vi "Refactor Classes in Project.vi"(8 "error in (no error)":errorcluster, 10 "rename data in":T1, 11 "project item in":refnum<vi>) -> (0 "error out":errorcluster, 2 "rename metadata out":T1, 3 "project item out":refnum<vi>, 4 "refactored overrides":T4[](array[typedef]), 6 "refactored classes":path[](array[path]))   [LabVIEW 2021, in "MeasurementService Editor.lvlib"]
uses:
  MeasurementService Editor.lvlib
  Rename Refactor Mapping Info.ctl
  Rename Refactor Data.ctl
  Refactor Dynamic Dispatch Member Result.ctl
  Rename String Mapping.ctl
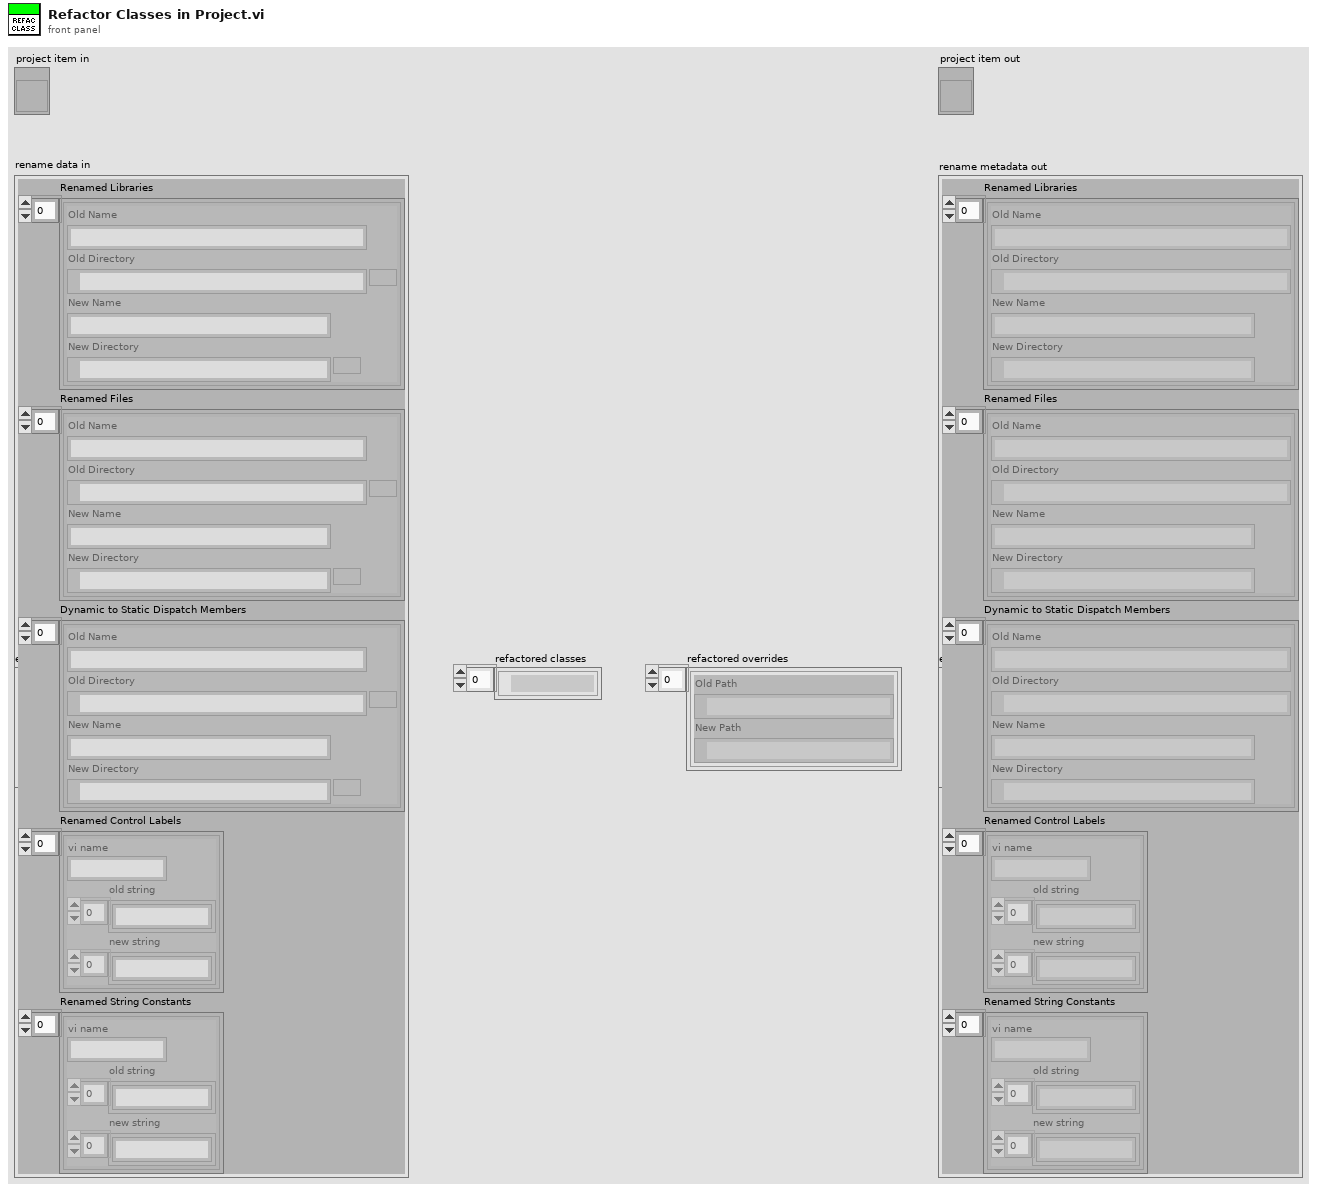
[diagram p1: front panel]
types:
  T1 = typedef "MeasurementService Editor.lvlib/Rename Refactor Data.ctl" = cluster{"Renamed Libraries":T2[], "Renamed Files":T2[], "Dynamic to Static Dispatch Members":T2[], "Renamed Control Labels":T3[], "Renamed String Constants":T3[]}
  T2 = typedef "MeasurementService Editor.lvlib/Rename Refactor Mapping Info.ctl" = cluster{"Old Name":string, "Old Directory":path, "New Name":string, "New Directory":path}
  T3 = typedef "MeasurementService Editor.lvlib/Rename String Mapping.ctl" = cluster{"vi name":string, "old string":string[], "new string":string[]}
  T4 = typedef "MeasurementService Editor.lvlib/Refactor Dynamic Dispatch Member Result.ctl" = cluster{"Old Path":path, "New Path":path}
  T5 = typedef "Copy of MeasurementService Editor.lvlib/Rename Refactor Data.ctl" = cluster{"Renamed Libraries":T6[], "Renamed Files":T6[], "Dynamic to Static Dispatch Members":T6[], "Renamed Control Labels":T7[], "Renamed String Constants":T7[]}
  T6 = typedef "Copy of MeasurementService Editor.lvlib/Rename Refactor Mapping Info.ctl" = cluster{"Old Name":string, "Old Directory":path, "New Name":string, "New Directory":path}
  T7 = typedef "Copy of MeasurementService Editor.lvlib/Rename String Mapping.ctl" = cluster{"vi name":string, "old string":string[], "new string":string[]}
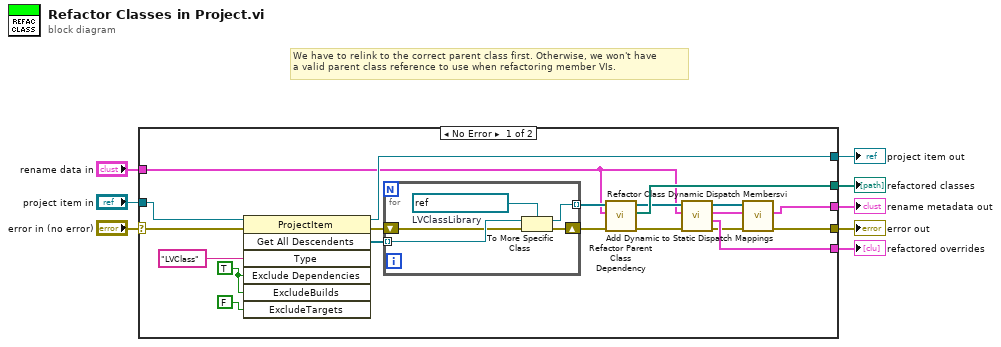
[diagram p0: block diagram]
diagram:
  # "We have to relink to the correct parent class first. Otherwise, we won't have\na valid parent class reference to use when refactoring member VIs."
  n1 = case shown="No Error" "error in (no error)" {
    selector: "error in (no error)" -> [w26 w36]
    tunnel: "project item in" -> [w28 w35]
    tunnel: [w27 w35] -> w7
    tunnel: [w12 w36] -> w6
    tunnel: "rename data in" -> [w15 w34]
    tunnel: [w18 _] -> w3
    tunnel: [w14 _] -> w2
    tunnel: [w10 w34] -> w1
    frame No Error {
      w25 = TRUE ("ExcludeDependencies")
      n2 = invoke class="ProjectItem" method="Get All Descendents"(reference=w28, error in=w26, "Type"="LVClass", "Exclude Dependencies"=w25, "ExcludeBuilds"=w25, "ExcludeTargets"=FALSE) -> (reference out=w27:refnum<vi>, error out=w21:errorcluster, "All Descendents"=w22:refnum<vi>[])  [unwired: 1 in, 4 out]
      n3 = for {
        tunnel: w22 -> [w33] mode=indexing
        shift-right: [w30] -> w20
        shift-left: w21 -> [w32]
        tunnel: [w29] -> w19 mode=indexing
        w31 = refnum<vi> refnum  # LVClassLibrary
        n4 = To More Specific Class(target class=w31, reference=w33, error in=w32) -> (specific class reference=w29:refnum<vi>, error out=w30:errorcluster)
      }
      n5 = call "Refactor Parent Class Dependency.vi"("error in (no error)"=w20, "rename data"=w15, "project classes in"=w19) -> ("error out"=w17:errorcluster, "refactored classes"=w18:path[], "project classes out"=w16:refnum<vi>[])  [unwired: 6 in]
      n6 = call "Refactor Class Dynamic Dispatch Membersvi.vi"("error in (no error)"=w17, "rename data in"=w15, "project classes in"=w16) -> ("error out"=w13:errorcluster, "refactor results"=w14:T4[], "rename metadata out"=w11:T1, "project classes out"=w9:refnum<vi>[])  [unwired: 5 in]
      n7 = call "Add Dynamic to Static Dispatch Mappings.vi"("error in (no error)"=w13, "rename data in"=w11, "project classes in"=w9) -> ("error out"=w12:errorcluster, "rename metadata out"=w10:T5)  [unwired: 6 in, 1 out]
    }
    frame Error {
    }
  }
  "project item out" <- w7
  "error out" <- w6
  "refactored classes" <- w3
  "refactored overrides" <- w2
  "rename metadata out" <- w1
